vi "Check If Inbounds.vi"(8 "error in (no error)":errorcluster, 11 "RDS Mission Controller Actor in":refnum<class "RDS Mission Controller Actor.lvclass">) -> (0 "error out":errorcluster, 3 "RDS Mission Controller Actor out":refnum<class "RDS Mission Controller Actor.lvclass">)   [LabVIEW 2015, in "RDS Mission Controller Actor.lvlib" / "RDS Mission Controller Actor.lvclass"]
uses:
  RDS Mission Controller Actor.lvclass
  RDS Mission Controller Actor.lvclass/RDS Mission Controller Actor.ctl
  Libraries/Geo/RDS Libraries.lvlib
panel:
  out "Bearing to Destination":dbl
  out "distance (m)":dbl
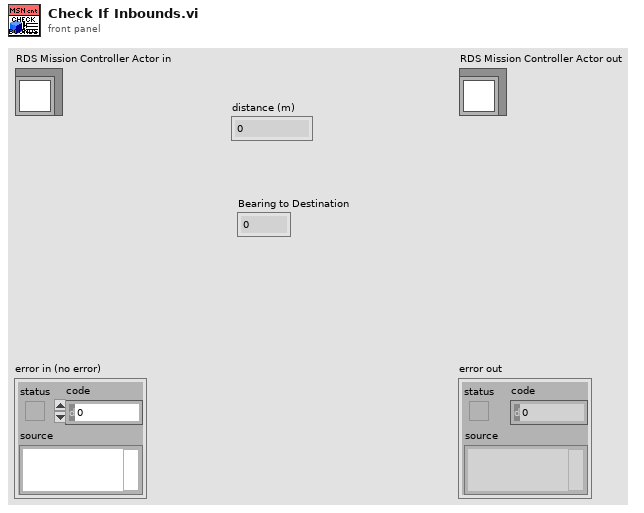
[diagram p1: front panel]
types:
  T1 = typedef "RDS Mission Controller Actor.lvlib/MissionOp.ctl" = cluster{"MissionOp Type":enum16{"Waypoint", "Loiter", "Wait", "Deploy AIP", "Stow AIP"}, "Duration (s)":u16, "Throttle":i16, "GPS Latitude":dbl, "GPS Longitude":dbl, "Loiter Range (m)":u16}
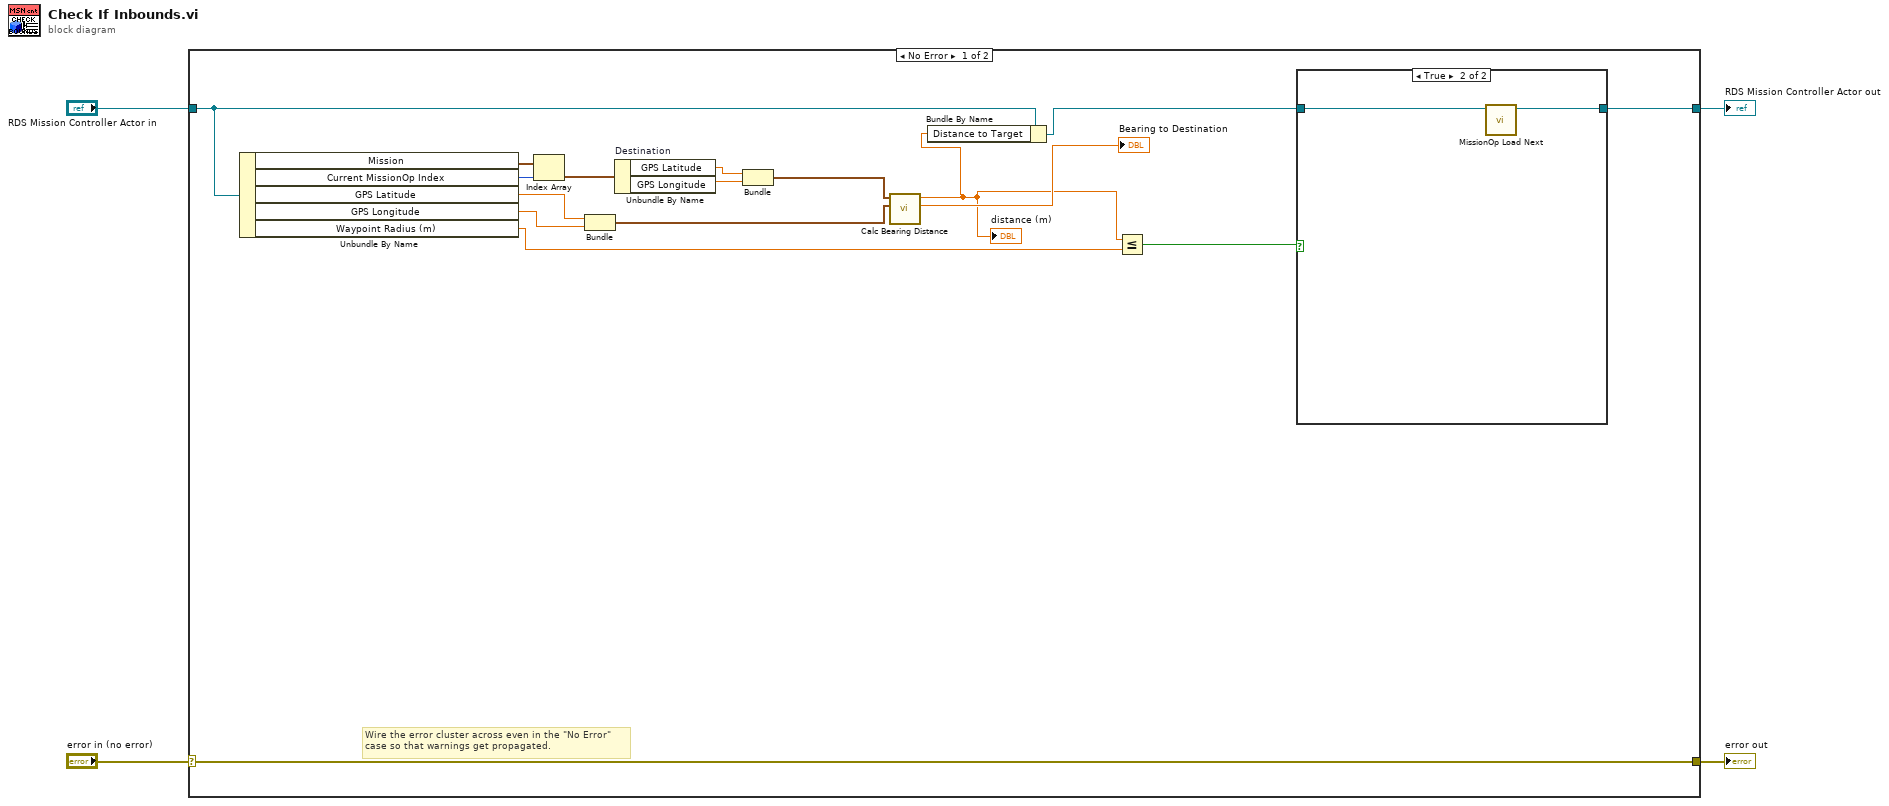
[diagram p0: block diagram]
diagram:
  n1 = case shown="No Error" "error in (no error)" {
    selector: "error in (no error)" -> [w21 w26]
    tunnel: [w21 w26] -> w3
    tunnel: [w8 w25] -> w1
    tunnel: "RDS Mission Controller Actor in" -> [w6 w25]
    frame No Error {
      # "Wire the error cluster across even in the \"No Error\"\ncase so that warnings get propagated."
      n2 = Unbundle By Name(w6) -> ("Mission"=w20:T1[], "Current MissionOp Index"=w19:i32, "GPS Latitude"=w14:ext, "GPS Longitude"=w13:ext, "Waypoint Radius (m)"=w10:dbl)
      n3 = Index Array(array=w20, index=w19) -> (element=w18:T1)
      n4 = Bundle("GPS Latitude"=w14, "GPS Longitude"=w13) -> (w12:cluster{"GPS Latitude":ext, "GPS Longitude":ext})  [unwired: 1 in]
      n5 = Unbundle By Name "Destination"(w18) -> ("GPS Latitude"=w17:dbl, "GPS Longitude"=w16:dbl)
      n6 = Bundle("GPS Latitude"=w17, "GPS Longitude"=w16) -> (w15:cluster{"GPS Latitude":dbl, "GPS Longitude":dbl})  [unwired: 1 in]
      n7 = call "Calc Bearing Distance.vi"("Current Location"=w12, "Destination"=w15) -> ("Bearing to Destination"=→"Bearing to Destination":dbl, "distance (m)"=w7:dbl)  [unwired: 8 in]
      "distance (m)" <- w7
      n8 = Bundle By Name(cluster=w6, "Distance to Target"=w7) -> (w5:refnum<class "RDS Mission Controller Actor.lvclass">)
      n9 = Less Or Equal?(x=w7, y=w10) -> (x <= y?=w9:bool)
      n10 = case shown="True" w9 {
        tunnel: [w22 w23] -> w8
        tunnel: w5 -> [w22 w24]
        frame False {
        }
        frame True {
          n11 = call "MissionOp Load Next.vi"("RDS Mission Controller Actor in"=w24) -> ("RDS Mission Controller Actor out"=w23:refnum<class "RDS Mission Controller Actor.lvclass">)  [unwired: 9 in, 1 out]
        }
      }
    }
    frame Error {
    }
  }
  "error out" <- w3
  "RDS Mission Controller Actor out" <- w1
